vi "Global variable_locations.vi"() -> ()   [LabVIEW 2016]
panel:
  out "Resynch_complete":bool
  in  "g_slack":dbl[](array[numeric])
  in  "b_slack":dbl[](array[numeric])
  in  "PV_comm_location":dbl[][](array[numeric])
  in  "Gen_comm_location":dbl[][](array[numeric])
  in  "BESS_comm_location":dbl[][](array[numeric])
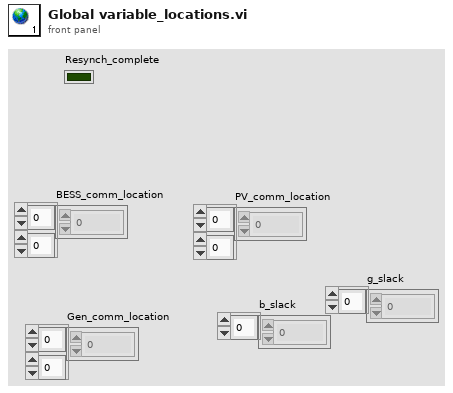
[diagram p1: front panel]
diagram:
